vi "Update Error.vi"(8 "error in (no error)":errorcluster, 9 "Stop Reason":T1, 10 "Received Error":errorcluster, 11 "Example Actor in":refnum<class "Example Actor.lvclass">) -> (0 "error out":errorcluster, 3 "Example Actor out":refnum<class "Example Actor.lvclass">)   [LabVIEW 2021, in "Example Iterator NR Actor Explicit Iteration.lvlib" / "Example Actor.lvclass"]
doc: "Displays the error received from the Iterator Actor."
uses:
  Example Actor.lvclass
  Abstract Iterator Actor/Stop Reason.ctl
  Example Actor.lvclass/Example Actor.ctl
  Abstract Iterator Actor/Abstract Iterator Actor.lvclass
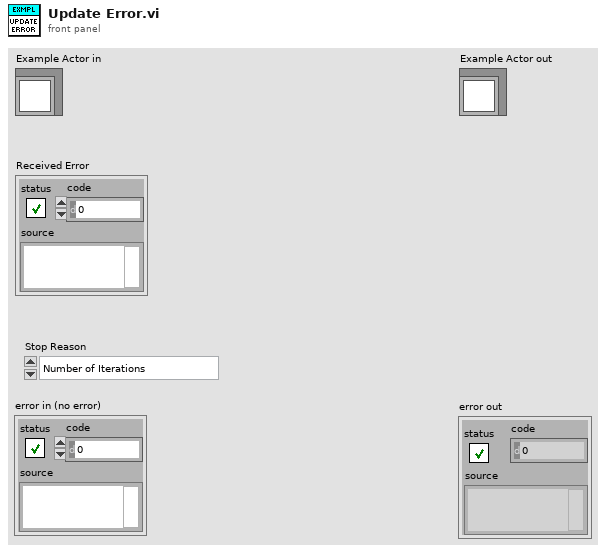
[diagram p1: front panel]
types:
  T1 = typedef "Iterator Actor.lvlib/Abstract Iterator Actor.lvclass/Stop Reason.ctl" = enum16{"Number of Iterations", "Time Elapsed", "Stopped Internally", "Stopped Externally"}
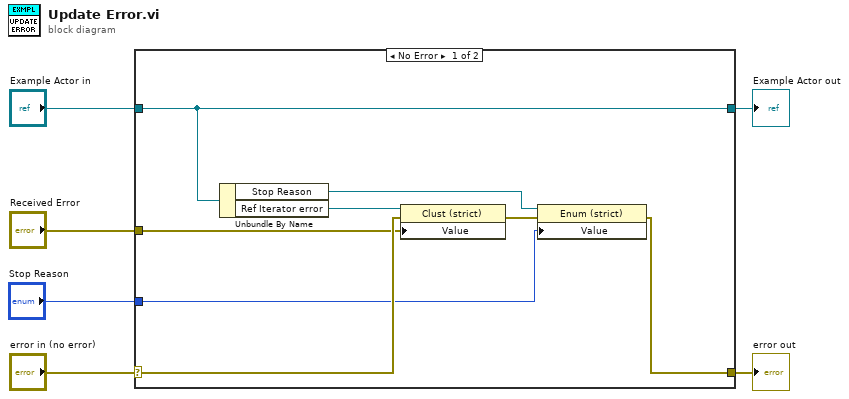
[diagram p0: block diagram]
diagram:
  n1 = case shown="No Error" "error in (no error)" {
    selector: "error in (no error)" -> [w12 w16]
    tunnel: [w7 w16] -> w5
    tunnel: [w14 w15] -> w3
    tunnel: "Example Actor in" -> [w14 w15]
    tunnel: "Received Error" -> [w11 _]
    tunnel: "Stop Reason" -> [w9 _]
    frame No Error {
      n2 = Unbundle By Name(w14) -> ("Stop Reason"=w10:refnum<vi>, "Ref Iterator error"=w13:refnum<vi>)
      n3 = property class="Clust (strict)"(reference=w13, error in=w12, "Value"=w11) -> (error out=w8:errorcluster)  [unwired: 1 out]
      n4 = property class="Enum (strict)"(reference=w10, error in=w8, "Value"=w9) -> (error out=w7:errorcluster)  [unwired: 1 out]
    }
    frame Error {
    }
  }
  "error out" <- w5
  "Example Actor out" <- w3
